vi "test_Create Message Group_Message Group created with desired Name.vi"(8 "error in (no error)":errorcluster, 11 "TestCase in":refnum<class "Instrument Addon Scripting API Messages Unit Tests.lvclass">) -> (0 "error out":errorcluster, 3 "TestCase out":refnum<class "Instrument Addon Scripting API Messages Unit Tests.lvclass">)   [LabVIEW 2023, in "Instrument Addon Scripting API Messages Unit Tests.lvclass"]
uses:
  Instrument Addon Scripting API Messages Unit Tests.lvclass
  Instrument Addon Scripting API Messages Unit Tests.lvclass/Instrument Addon Scripting API Messages Unit Tests.ctl
  Addon/Addon Shared/SubVIs/Constants.vi
  NationalInstruments.VeriStand.SystemDefinitionAPI
  <vilib>/addons/_JKI Toolkits/VI Tester/TestCase.llb/TestCase.lvclass
  Addon/Addon Shared/Instrument Addon Shared.lvlib
  <vilib>/NI VeriStand/Custom Device API/Custom Device API.lvlib
  APIs/Scripting API/Instrument Addon Scripting API.lvlib
  C:/Program Files/National Instruments/LabVIEW 2024/vi.lib/addons/_JKI Toolkits/VI Tester/TestCase.llb/TestCase.lvclass
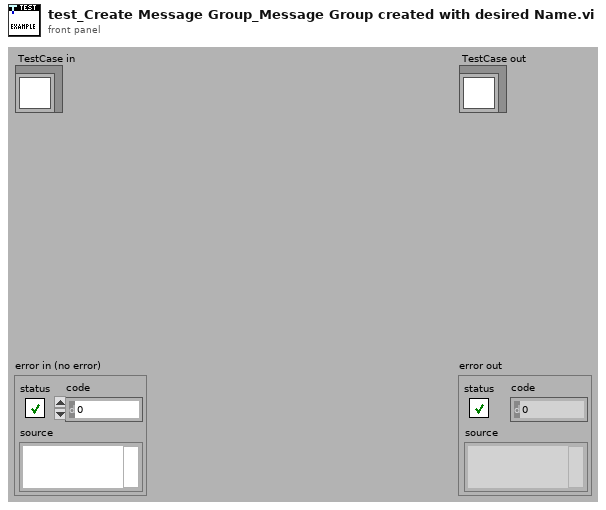
[diagram p1: front panel]
types:
  T1 = typedef "Custom Device API.lvlib/Custom Device Item Ref.ctl" = u64
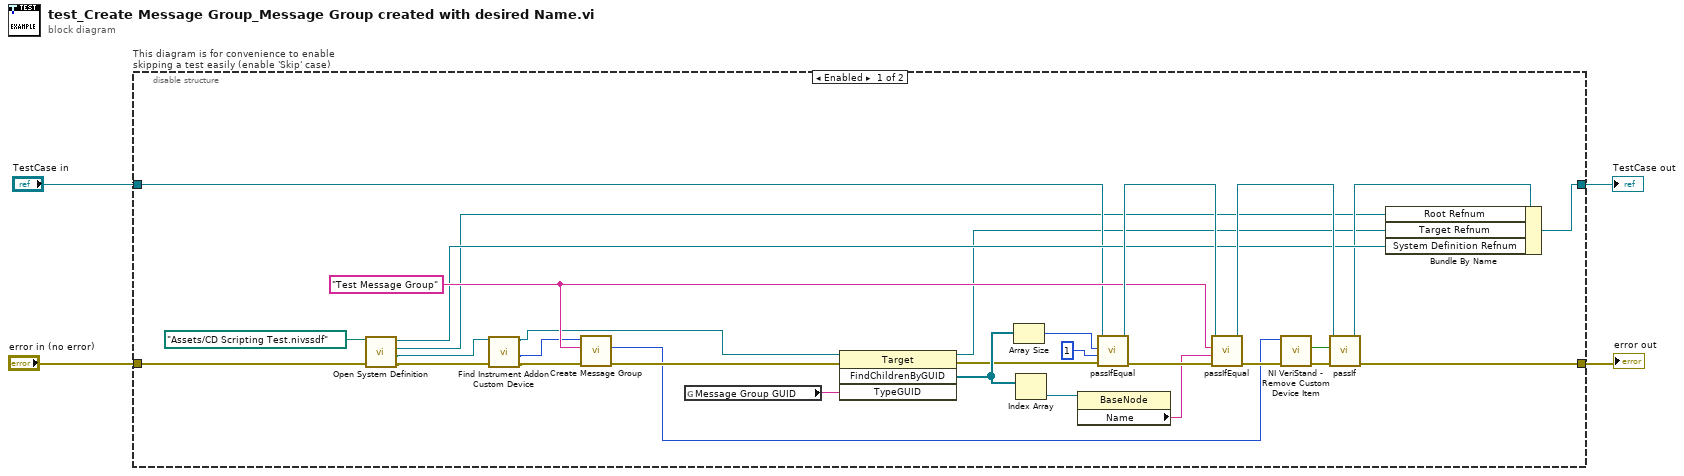
[diagram p0: block diagram]
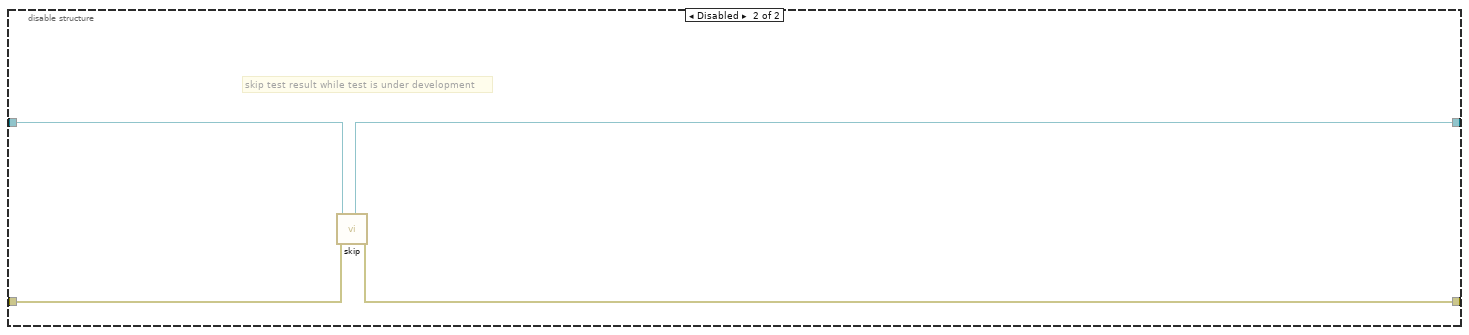
[diagram p2: hidden frame]
diagram:
  n1 = disable-structure "This diagram is for convenience to enable skipping a test easily (enable 'Skip' case)" shown="Enabled" {
    disable-tunnel: "TestCase in" -> [w9 w38]
    disable-tunnel: [w7 w36] -> w1
    disable-tunnel: [w24 w37] -> w3
    disable-tunnel: "error in (no error)" -> [w18 w35]
    frame Enabled {
      w21 = "Test Message Group" ("Section Name")
      n2 = call "Open System Definition.vi"("error in (no error)"=w18, "System Definition File"=path "Assets/CD Scripting Test.nivssdf" ("SDF file")) -> ("error out"=w14:errorcluster, "Target Refnum"=w15:refnum<k24>, "Root Refnum"=w5:refnum<k24>, "System Definition Refnum"=w16:refnum<k24>)  [unwired: 6 in]
      n3 = call "Find Instrument Addon Custom Device.vi"("error in"=w14, "target in"=w15) -> ("error out"=w11:errorcluster, "NodeID"=w12:u64, "target out"=w13:refnum<k24>)  [unwired: 7 in]
      n4 = call "Create Message Group.vi"("error in (no error)"=w11, "message group name"=w21, "instrument addon refnum in"=w12) -> ("error out"=w20:errorcluster, "message group refnum out"=w19:T1)  [unwired: 6 in, 1 out]
      n5 = global read "Constants.vi" "Message Group GUID"() -> (w34:string)
      n6 = invoke class="Target" method="FindChildrenByGUID"(reference=w13, error in=w20, "TypeGUID"=w34) -> (reference out=w6:refnum<k24>, error out=w10:errorcluster, "FindChildrenByGUID"=w33:refnum<k24>[])  [unwired: 1 in, 1 out]
      n7 = Array Size(array=w33) -> (size(s)=w32:i32)
      n8 = Index Array(array=w33) -> (element=w27:refnum<k24>)  [unwired: 1 in]
      n9 = property class="BaseNode"(reference=w27) -> ("Name"=w28:string)  [unwired: 1 in, 2 out]
      n10 = call-dynamic "passIfEqual.vi"("error in (no error)"=w10, "y"=1 ("size(s)"), "x"=w32, "TestCase in"=w9) -> ("error out"=w30:errorcluster, "TestCase out"=w29:refnum<class "Instrument Addon Scripting API Messages Unit Tests.lvclass">)  [unwired: 6 in]
      n11 = call-dynamic "passIfEqual.vi"("error in (no error)"=w30, "y"=w28, "x"=w21, "TestCase in"=w29) -> ("error out"=w26:errorcluster, "TestCase out"=w22:refnum<class "Instrument Addon Scripting API Messages Unit Tests.lvclass">)  [unwired: 6 in]
      n12 = call <vilib>:"NI VeriStand - Remove Custom Device Item.vi"("error in (no error)"=w26, "Item Ref in"=w19) -> ("error out"=w25:errorcluster, "Deleted?"=w23:bool)  [unwired: 8 in]
      n13 = call-dynamic "passIf.vi"("error in (no error)"=w25, "pass"=w23, "TestCase in"=w22) -> ("error out"=w24:errorcluster, "TestCase out"=w8:refnum<class "Instrument Addon Scripting API Messages Unit Tests.lvclass">)  [unwired: 7 in]
      n14 = Bundle By Name(cluster=w8, "Root Refnum"=w5, "Target Refnum"=w6, "System Definition Refnum"=w16) -> (w7:refnum<class "Instrument Addon Scripting API Messages Unit Tests.lvclass">)
    }
    frame Disabled {
      # "skip test result while test is under development"
      n15 = call <vilib>:"skip.vi"("error in (no error)"=w35, "TestCase in"=w38) -> ("error out"=w37:errorcluster, "TestCase out"=w36:refnum<class "Instrument Addon Scripting API Messages Unit Tests.lvclass">)  [unwired: 8 in]
    }
  }
  "error out" <- w3
  "TestCase out" <- w1
